vi "Parse Setting file.vi"(8 "error in (no error)":errorcluster, 11 "Setring file path":path) -> (0 "error out":errorcluster, 1 "MAC":string, 2 "SN":string, 3 "Action":i32)   [LabVIEW 2012]
panel:
  out "text":string
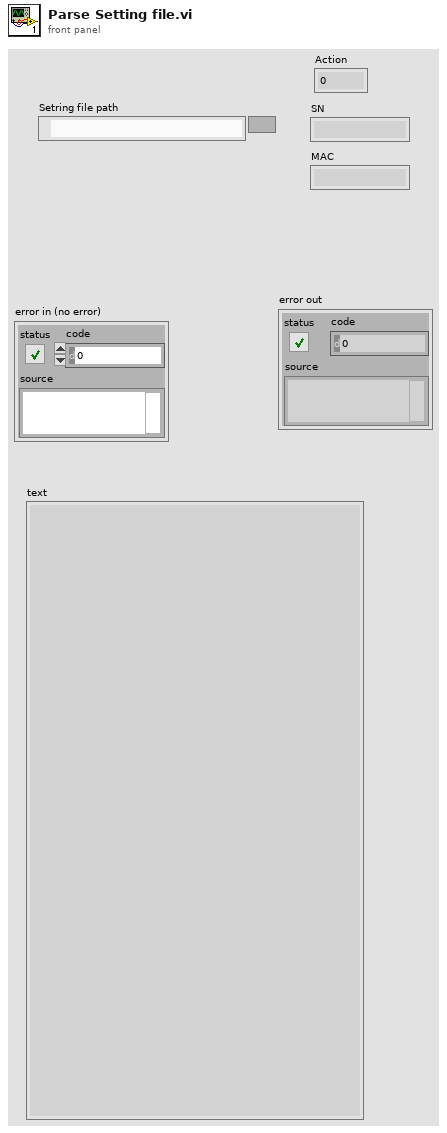
[diagram p1: front panel]
types:
  T1 = enum16{"open", "replace", "create", "open or create", "replace or create", "replace or create with confirmation"}
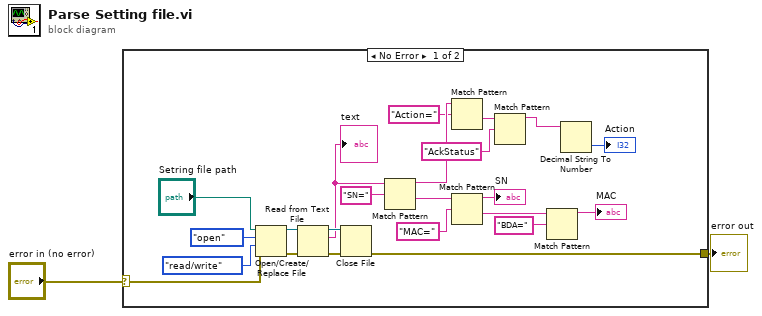
[diagram p0: block diagram]
diagram:
  n1 = case shown="No Error" "error in (no error)" {
    selector: "error in (no error)" -> [w6 _]
    tunnel: [w5 _] -> w1
    frame No Error {
      n2 = Open/Create/Replace File(file path (use dialog)="Setring file path", error in=w6, operation (0:open)=T1."open", access (0:read/write)=enum16{"read/write", "read-only", "write-only"}."read/write") -> (refnum out=w22:refnum<file>, error out=w12:errorcluster)  [unwired: 2 in, 1 out]
      n3 = Read from Text File(file (use dialog)=w22, error in=w12) -> (refnum out=w21:refnum<file>, text=w20:string, error out=w11:errorcluster)  [unwired: 2 in, 1 out]
      "text" <- w20
      n4 = Close File(refnum=w21, error in=w11) -> (error out=w5:errorcluster)  [unwired: 1 out]
      n5 = Match Pattern(string=w20, regular expression="SN=") -> (before substring=w10:string, after substring=w16:string)  [unwired: 1 in, 2 out]
      n6 = Match Pattern(string=w10, regular expression="Action=") -> (after substring=w8:string)  [unwired: 1 in, 3 out]
      n7 = Match Pattern(string=w16, regular expression="MAC=") -> (before substring=→"SN":string, after substring=w15:string)  [unwired: 1 in, 2 out]
      n8 = Match Pattern(string=w8, regular expression="AckStatus") -> (before substring=w4:string)  [unwired: 1 in, 3 out]
      n9 = Match Pattern(string=w15, regular expression="BDA=") -> (before substring=→"MAC":string)  [unwired: 1 in, 3 out]
      n10 = Decimal String To Number(string=w4) -> (number=→"Action":i32)  [unwired: 2 in, 1 out]
    }
    frame Error {
    }
  }
  "error out" <- w1
